vi "denoise_filter.vi"(3 "Filter Level":i32, 4 "Signal Input":bool) -> (1 "Signal Output":bool)   [LabVIEW 2020]
panel:
  out "Post-Filter":i16(graph)
  out "Pre-Filter":i16(graph)
  # "Leave these as is, they are for the wire input and output for\nthe sub-vi"
  # "Change this to be the number of points that you want to check\nfor the filter"
  # "Two charts for a sid-by-side comparison to make sure that the signal is being filtered enough"
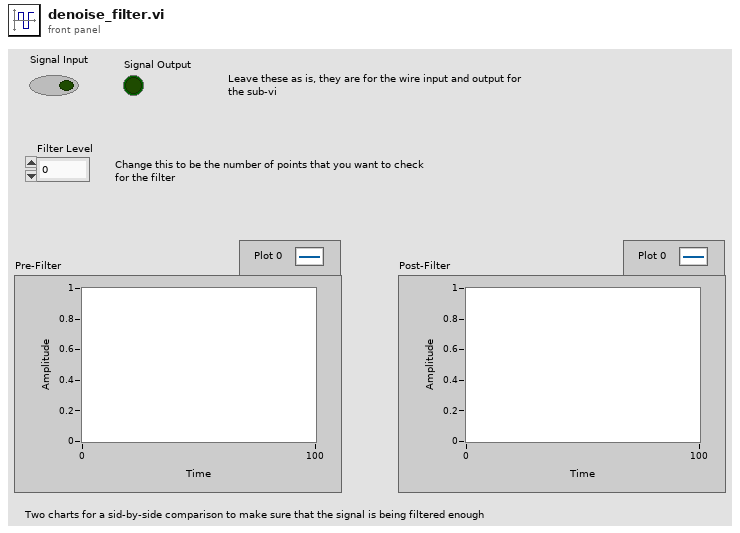
[diagram p1: front panel]
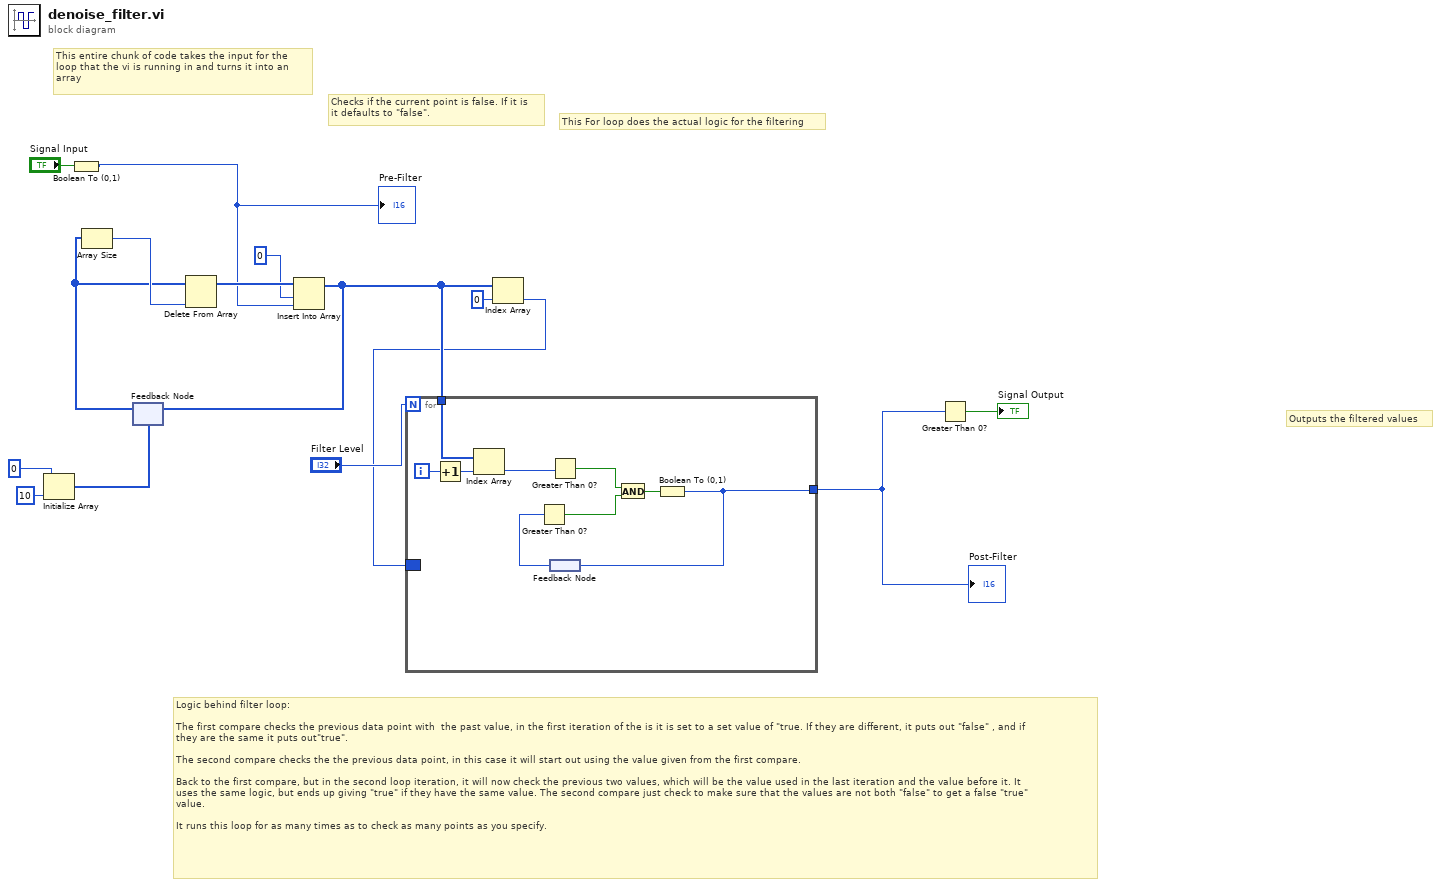
[diagram p0: block diagram]
diagram:
  # "Logic behind filter loop:\n\nThe first compare checks the previous data point with  the past value, in the first iteration of the is it is set to a set value of \"true. If they are different, it puts out \"false\" , and if \nthey are the same it puts out\"true\".\n\nThe second compare checks the the previous data point, in this case it will start out using the value given from the first compare.\n\nBack to the first compare, but in the second loop iteration, it will now check the previous two values, which will be the value used in the last iteration and the value before it. It \nuses the same logic, but ends up giving \"true\" if they have the same value. The second compare just check to make sure that the values are not both \"false\" to get a false \"true\"\nvalue.\n\nIt runs this loop for as many times as to check as many points as you specify."
  # "Checks if the current point is false. If it is\nit defaults to \"false\"."
  # "Outputs the filtered values"
  # "This entire chunk of code takes the input for the\nloop that the vi is running in and turns it into an \narray"
  # "This For loop does the actual logic for the filtering"
  n1 = Initialize Array(i16 0 ("element"), 10 ("dimension size")) -> (w4:i16[])
  n2 = Boolean To (0,1)(Boolean="Signal Input") -> (0, 1=w5:i16)
  "Pre-Filter" <- w5
  n3 = feedback #1(w4) -> (w12:i16[])
  n4 = Array Size(array=w12) -> (size(s)=w13:i32)
  n5 = Delete From Array(array=w12, index=w13) -> (array with subset deleted=w11:i16[])  [unwired: 1 in, 1 out]
  n6 = Insert Into Array(array=w11, index=0, new element=w5) -> (w7:i16[])
  n7 = feedback-in #1(w7) -> ()
  n8 = Index Array(array=w7, index=0) -> (element=w3:i16)
  n9 = for {
    N: "Filter Level" -> [_]
    tunnel: w7 -> [w24]
    border: w3 -> [_]
    tunnel: [w16] -> w1
    i -> [w23]
    n10 = Increment(x=w23) -> (x+1=w22:i32)
    n11 = Index Array(array=w24, index=w22) -> (element=w21:i16)
    n12 = Greater Than 0?(x=w21) -> (x > 0?=w19:bool)
    n13 = feedback #2() -> (w18:i16)
    n14 = Greater Than 0?(x=w18) -> (x > 0?=w20:bool)
    n15 = And(x=w19, y=w20) -> (x .and. y?=w17:bool)
    n16 = Boolean To (0,1)(Boolean=w17) -> (0, 1=w16:i16)
    n17 = feedback-in #2(w16) -> ()
  }
  "Post-Filter" <- w1
  n18 = Greater Than 0?(x=w1) -> (x > 0?=→"Signal Output":bool)
